vi "StartRecordSpecialMarlin.vi"(4 "error in (no error)":errorcluster, 6 "ClusterRefCtrlIN":T1, 7 "task/channels in":refnum<k21>) -> (0 "error out":errorcluster, 2 "RecStarted":bool, 3 "task out":refnum<k21>)   [LabVIEW 2015]
uses:
  DefDeType/ClusterRefCtrl.ctl
  <vilib>/DAQmx/write.llb/DAQmx Write (Digital Bool 1Line 1Point).vi
  <vilib>/DAQmx/miscellaneous.llb/DAQmx Fill In Error Info.vi
  Globals/NortekInstruction.vi
  Globals/QualisysInstruction.vi
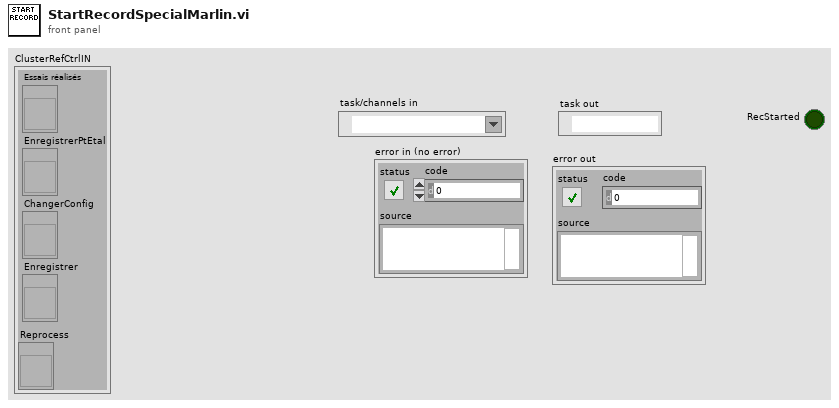
[diagram p1: front panel]
types:
  T1 = typedef "ClusterRefCtrl.ctl" = cluster{"Essais réalisés":refnum<vi>, "EnregistrerPtEtal":refnum<vi>, "ChangerConfig":refnum<vi>, "Enregistrer":refnum<vi>, "Reprocess":refnum<vi>}
  T2 = enum8{"Enabled", "Disabled", "Disabled and Grayed Out"}
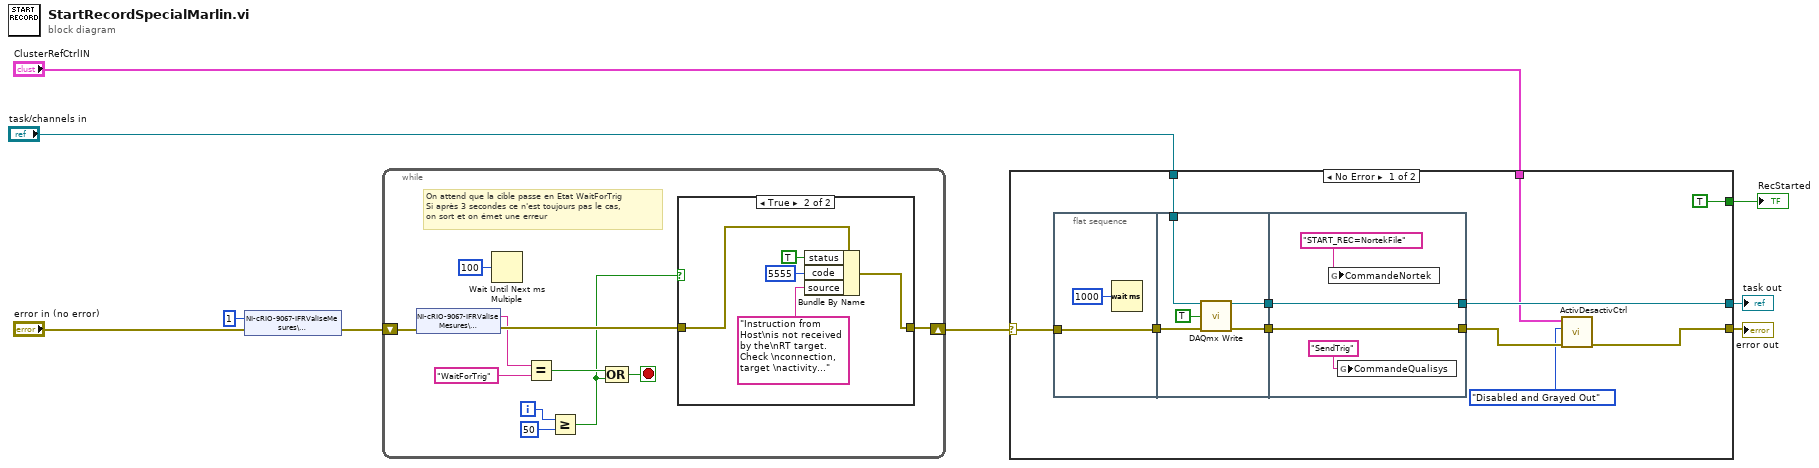
[diagram p0: block diagram]
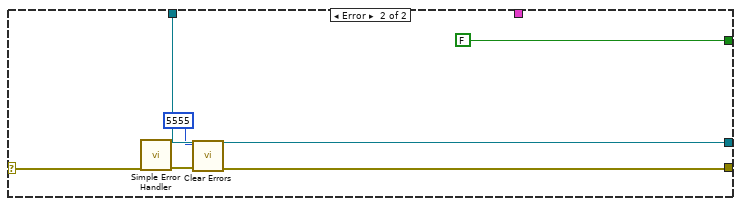
[diagram p2: hidden frame]
diagram:
  n1 = shared-variable "NI-cRIO-9067-IFRValiseMesures\\Bibliothèque2Variables.lvlib\\Instruction"(u8 1 ("Instruction"), error in="error in (no error)") -> (error out=w7:errorcluster)
  n2 = while {
    shift-right: [w11] -> w6
    shift-left: w7 -> [w20]
    i -> [w17]
    stop <- w14 stop-if-true
    # "On attend que la cible passe en Etat WaitForTrig\nSi après 3 secondes ce n'est toujours pas le cas, \non sort et on émet une erreur"
    n3 = shared-variable "NI-cRIO-9067-IFRValiseMesures\\Bibliothèque2Variables.lvlib\\RTState"(error in=w20) -> (w10:string, error out=w13:errorcluster)
    n4 = Wait Until Next ms Multiple(millisecond multiple=u32 100) -> ()  [unwired: 1 out]
    n5 = Equal?(x=w10, y="WaitForTrig") -> (x = y?=w15:bool)
    n6 = Greater Or Equal?(x=w17, y=50) -> (x >= y?=w12:bool)
    n7 = Compound Arithmetic op=OR(w15, w12) -> (w14:bool)
    n8 = case shown="True" w12 {
      tunnel: w13 -> [w21 w26]
      tunnel: [w21 w22] -> w11
      frame False {
      }
      frame True {
        n9 = Bundle By Name(cluster=w26, "status"=TRUE, "code"=5555, "source"="Instruction from Host\nis not received by the\nRT target. Check \nconnection, target \nactivity...") -> (w22:errorcluster)
      }
    }
  }
  n10 = case shown="No Error" w6 {
    selector: w6 -> [w37 w53]
    tunnel: "task/channels in" -> [w35 w54]
    tunnel: [w31 w50] -> w3
    tunnel: [w34 w54] -> w4
    tunnel: [TRUE ("RecStarted") FALSE ("RecStarted")] -> w2
    tunnel: "ClusterRefCtrlIN" -> [w30 _]
    frame No Error {
      n11 = flat-sequence {
        tunnel: w37 -> [w38]
        tunnel: [w38] -> w36
        tunnel: w36 -> [w43]
        tunnel: w35 -> [w41]
        tunnel: [w42] -> w28
        tunnel: [w40] -> w27
        tunnel: [w47] -> w34
        tunnel: [w48] -> w32
        tunnel: w28 -> [w48]
        tunnel: w27 -> [w47]
        frame #0 {
          n12 = Wait (ms)(milliseconds to wait=u32 1000) -> ()  [unwired: 1 out]
        }
        frame #1 {
          n13 = call-poly <vilib>:"DAQmx Write.vi"("task/channels in"=w41, "data"=TRUE, "error in"=w43) -> ("task out"=w40:refnum<k21>, "error out"=w42:errorcluster)  [unwired: 10 in, 1 out]
        }
        frame #2 {
          n14 = global write "NortekInstruction.vi" "CommandeNortek"("START_REC=NortekFile" ("Command")) -> ()
          n15 = global write "QualisysInstruction.vi" "CommandeQualisys"("SendTrig" ("Command")) -> ()
        }
      }
      n16 = call "ActivDesactivCtrl.vi"("error in (no error)"=w32, "Disabled"=T2."Disabled and Grayed Out", "Cluster"=w30) -> ("error out"=w31:errorcluster)  [unwired: 4 in]
    }
    frame Error {
      n17 = call <vilib>:"Simple Error Handler.vi"("error in (no error)"=w53) -> ("error out"=w52:errorcluster)  [unwired: 4 in, 4 out]
      n18 = call <vilib>:"Clear Errors.vi"("error in (no error)"=w52, "specific error code to clear (0: all)"=5555) -> ("error out"=w50:errorcluster)  [unwired: 4 in, 1 out]
    }
  }
  "task out" <- w4
  "error out" <- w3
  "RecStarted" <- w2
